vi "Property Test.vi"() -> ()   [LabVIEW 2015]
uses:
  <vilib>/_script/All Supported PropertiesOrMethods TypeDefs/ASPM_ArrayOfUniqueIDStringDatanameShortnameLongname.ctl
  <vilib>/_script/All Supported PropertiesOrMethods TypeDefs/ASPM_UniqueIDStringDatanameShortnameLongname.ctl
  <vilib>/Erdos Miller/LV-Scripting/LV-Scripting.lvlib
panel:
  out "Properties[]":T1
  out "Class Name":string
  in  "Tab Control":enum32{"Page 1", "Page 2"}(tab)
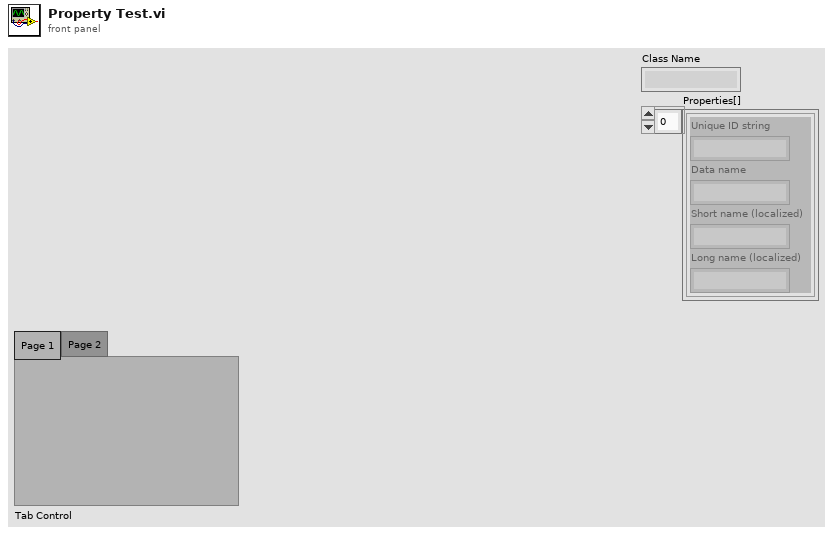
[diagram p1: front panel]
types:
  T1 = typedef "ASPM_ArrayOfUniqueIDStringDatanameShortnameLongname.ctl" = T2[]
  T2 = typedef "ASPM_UniqueIDStringDatanameShortnameLongname.ctl" = cluster{"Unique ID string":string, "Data name":string, "Short name (localized)":string, "Long name (localized)":string}
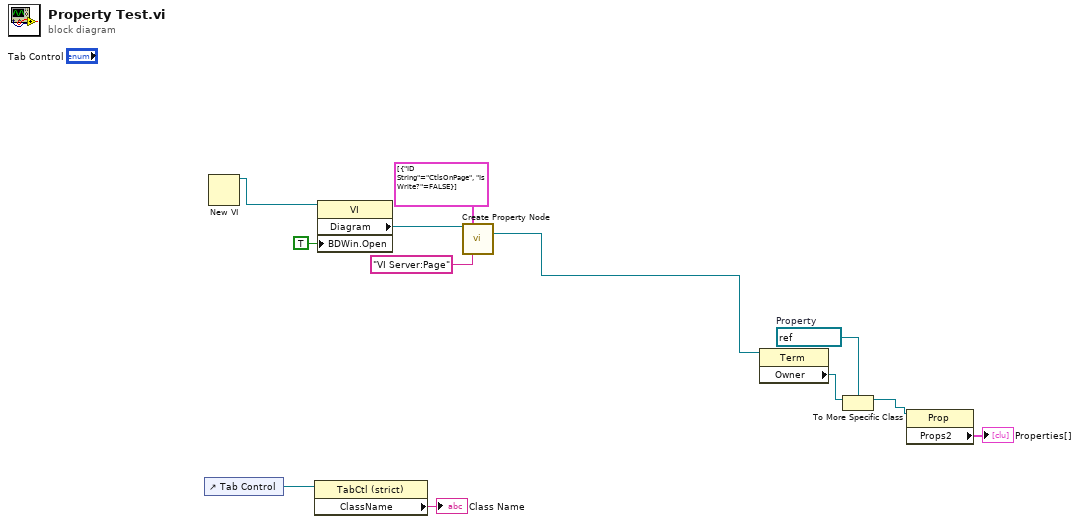
[diagram p0: block diagram]
diagram:
  w3 = refnum<vi> refnum  # Property
  n1 = control-ref of="Tab Control"() -> (w7:refnum<vi>)
  n2 = New VI() -> (3:w12:refnum<vi>)  [unwired: 7 in, 1 out]
  n3 = property class="TabCtl (strict)"(reference=w7) -> ("ClassName"=→"Class Name":string)  [unwired: 1 in, 2 out]
  n4 = property class="VI"(reference=w12, "BDWin.Open"=TRUE ("Block Diagram Window:Open")) -> ("Diagram"=w10:refnum<vi>)  [unwired: 1 in, 2 out]
  n5 = call <vilib>:"Create Property Node.vi"("Diagram in"=w10, "Properties"=cluster{"ID String":string, "Is Write?":bool}[] [{"ID String"="CtlsOnPage", "Is Write?"=FALSE}], "Class Name"="VI Server:Page") -> ("reference out"=w5:refnum<vi>)  [unwired: 8 in, 4 out]
  n6 = property class="Term"(reference=w5) -> ("Owner"=w4:refnum<vi>)  [unwired: 1 in, 2 out]
  n7 = To More Specific Class(target class=w3, reference=w4) -> (specific class reference=w2:refnum<vi>)  [unwired: 1 in, 1 out]
  n8 = property class="Prop"(reference=w2) -> ("Props2"=→"Properties[]":T1)  [unwired: 1 in, 2 out]
